vi "Get Element References.vi"(8 "error in (no error)":errorcluster, 11 "Filled Text Fields Actor in":refnum<class "Filled Text Fields Actor.lvclass">) -> (0 "error out":errorcluster, 3 "Filled Text Fields Actor out":refnum<class "Filled Text Fields Actor.lvclass">)   [LabVIEW 2017, in "Filled Text Fields Actor.lvlib" / "Filled Text Fields Actor.lvclass"]
uses:
  Filled Text Fields Actor.lvclass
  Filled Text Fields Actor.lvclass/Filled Text Fields Actor.ctl
  <vilib>/UserTags/UserTags.lvlib
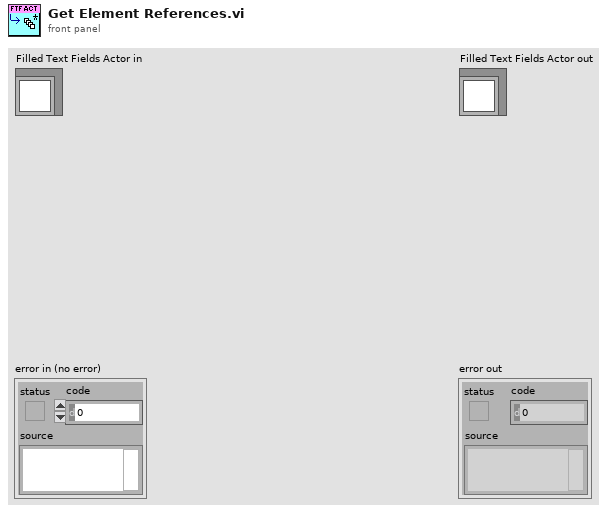
[diagram p1: front panel]
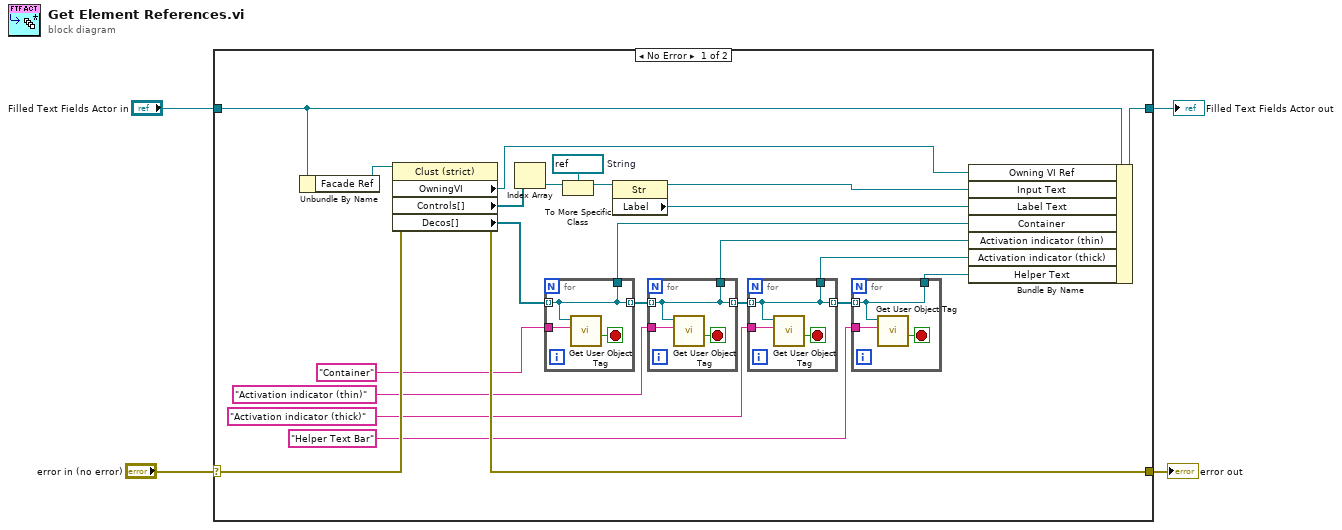
[diagram p0: block diagram]
diagram:
  n1 = case shown="No Error" "error in (no error)" {
    selector: "error in (no error)" -> [w28 w42]
    tunnel: [w27 w42] -> w3
    tunnel: [w18 w41] -> w1
    tunnel: "Filled Text Fields Actor in" -> [w20 w41]
    frame No Error {
      w22 = refnum<vi> refnum  # String
      n2 = Unbundle By Name(w20) -> ("Facade Ref"=w19:refnum<vi>)
      n3 = property class="Clust (strict)"(reference=w19, error in=w28) -> (error out=w27:errorcluster, "OwningVI"=w5:refnum<vi>, "Controls[]"=w24:refnum<vi>[], "Decos[]"=w25:refnum<vi>[])  [unwired: 1 out]
      n4 = Index Array(array=w24) -> (element=w23:refnum<vi>)  [unwired: 1 in]
      n5 = for {
        tunnel: w25 -> [w38] mode=indexing
        tunnel: "Container" ("Tag Name") -> [w40]
        tunnel: [w38] -> w15
        tunnel: [w38] -> w14 mode=indexing
        stop <- w39 stop-if-true
        n6 = call <vilib>:"Get User Object Tag.vi"("Tag Name"=w40, "Generic Refnum"=w38) -> ("Was Tag Found?"=w39:bool)  [unwired: 6 in, 3 out]
      }
      n7 = To More Specific Class(target class=w22, reference=w23) -> (specific class reference=w21:refnum<vi>)  [unwired: 1 in, 1 out]
      n8 = property class="Str"(reference=w21) -> (reference out=w17:refnum<vi>, "Label"=w16:refnum<vi>)  [unwired: 1 in, 1 out]
      n9 = for {
        tunnel: w14 -> [w35] mode=indexing
        tunnel: "Activation indicator (thin)" ("Tag Name") -> [w37]
        tunnel: [w35] -> w10
        tunnel: [w35] -> w13 mode=indexing
        stop <- w36 stop-if-true
        n10 = call <vilib>:"Get User Object Tag.vi"("Tag Name"=w37, "Generic Refnum"=w35) -> ("Was Tag Found?"=w36:bool)  [unwired: 6 in, 3 out]
      }
      n11 = for {
        tunnel: w13 -> [w32] mode=indexing
        tunnel: "Activation indicator (thick)" ("Tag Name") -> [w34]
        tunnel: [w32] -> w11
        tunnel: [w32] -> w9 mode=indexing
        stop <- w33 stop-if-true
        n12 = call <vilib>:"Get User Object Tag.vi"("Tag Name"=w34, "Generic Refnum"=w32) -> ("Was Tag Found?"=w33:bool)  [unwired: 6 in, 3 out]
      }
      n13 = for {
        tunnel: w9 -> [w29] mode=indexing
        tunnel: "Helper Text Bar" ("Tag Name") -> [w31]
        tunnel: [w29] -> w12
        stop <- w30 stop-if-true
        n14 = call <vilib>:"Get User Object Tag.vi"("Tag Name"=w31, "Generic Refnum"=w29) -> ("Was Tag Found?"=w30:bool)  [unwired: 6 in, 3 out]
      }
      n15 = Bundle By Name(cluster=w20, "Owning VI Ref"=w5, "Input Text"=w17, "Label Text"=w16, "Container"=w15, "Activation indicator (thin)"=w10, "Activation indicator (thick)"=w11, "Helper Text"=w12) -> (w18:refnum<class "Filled Text Fields Actor.lvclass">)
    }
    frame Error {
    }
  }
  "error out" <- w3
  "Filled Text Fields Actor out" <- w1
